vi "EnqueData.vi"(8 "error in (no error)":errorcluster, 11 "DataReceiver in":refnum<class "DataReceiver.lvclass">) -> (0 "error out":errorcluster, 3 "DataReceiver out":refnum<class "DataReceiver.lvclass">)   [LabVIEW 2010, in "DataReceiver.lvclass"]
uses:
  DataReceiver.lvclass
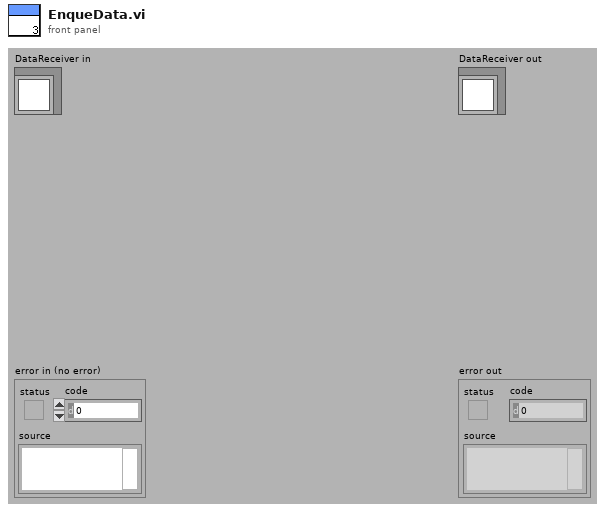
[diagram p1: front panel]
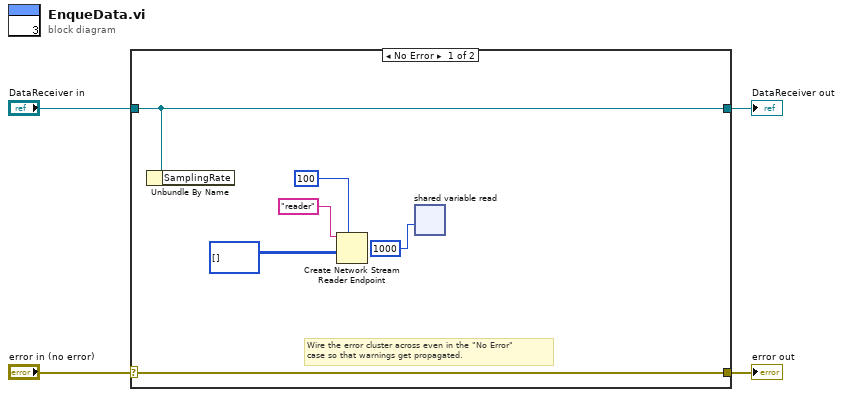
[diagram p0: block diagram]
diagram:
  n1 = case shown="No Error" "error in (no error)" {
    selector: "error in (no error)" -> [w10 w12]
    tunnel: [w10 w12] -> w3
    tunnel: [w5 w11] -> w1
    tunnel: "DataReceiver in" -> [w5 w11]
    frame No Error {
      # "Wire the error cluster across even in the \"No Error\"\ncase so that warnings get propagated."
      n2 = Unbundle By Name(w5) -> ()  [unwired: 1 out]
      n3 = Create Network Stream Reader Endpoint(7:100 ("reader buffer size"), 9:i32[][] [], 11:"reader" ("writer name")) -> ()  [unwired: 3 in, 2 out]
      n4 = shared-variable-read(1000 ("timeout in ms (-1)")) -> ()  [unwired: 3 in, 4 out]
    }
    frame Error {
    }
  }
  "error out" <- w3
  "DataReceiver out" <- w1
